vi "Dynamic call-Functional Viewer Window.vi"(8 "error in (no error)":errorcluster, 11 "Experiment data folder path":path) -> ()   [LabVIEW 2017]
uses:
  Globals/gl_Funct imaging UI.vi
panel:
  out "path":path
  # "Calls the \"Functional Viewer\" window dynamically."
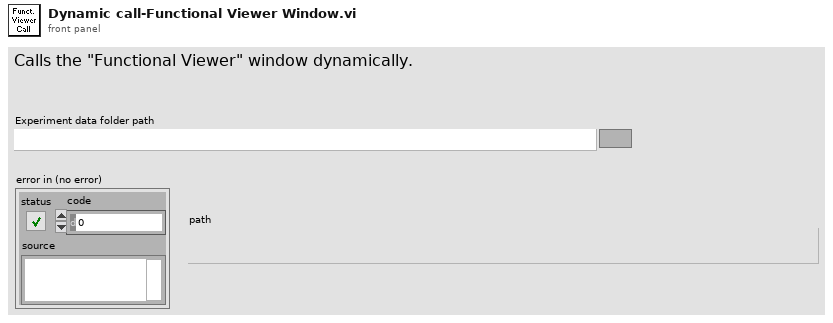
[diagram p1: front panel]
types:
  T1 = enum16{"Register", "Load dataset in funct viewer", "Re-process data"}
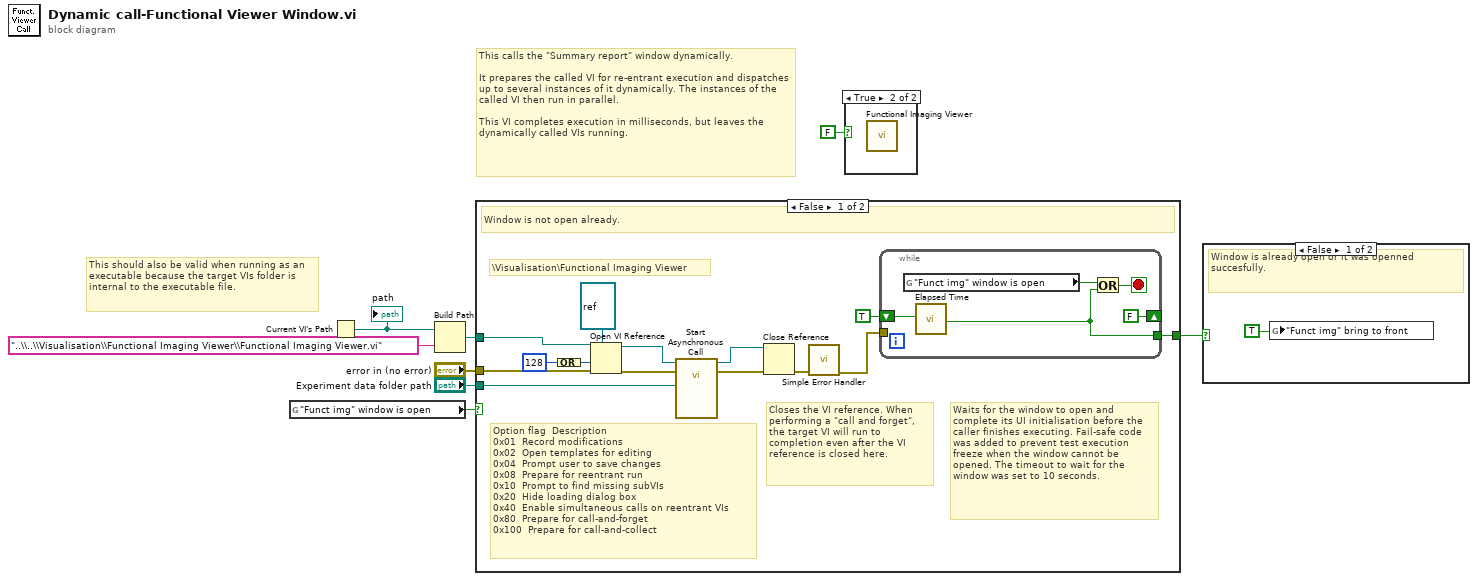
[diagram p0: block diagram]
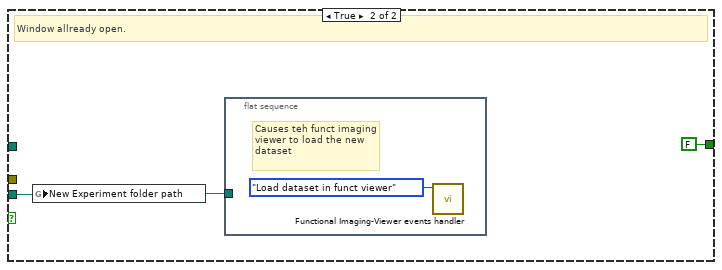
[diagram p4: hidden frame]
diagram:
  # "This should also be valid when running as an executable because the target VIs folder is internal to the executable file."
  # "This calls the \"Summary report\" window dynamically.\n\nIt prepares the called VI for re-entrant execution and dispatches up to several instances of it dynamically. The instances of the called VI then run in parallel.\n\nThis VI completes execution in milliseconds, but leaves the dynamically called VIs running."
  n1 = global read "gl_Funct imaging UI.vi" "\"Funct img\" window is open"() -> (w8:bool)
  n2 = Current VI's Path() -> (path=w4:path)
  "path" <- w4
  n3 = Build Path(base path=w4, name or relative path="..\\..\\Visualisation\\Functional Imaging Viewer\\Functional Imaging Viewer.vi") -> (appended path=w3:path)
  n4 = case shown="False" w8 {
    tunnel: "Experiment data folder path" -> [w12 w28]
    tunnel: "error in (no error)" -> [w11 _]
    tunnel: w3 -> [w10 _]
    tunnel: [w9 FALSE ("Time has Elapsed")] -> w1
    frame False {
      # "\\Visualisation\\Functional Imaging Viewer"
      # "Waits for the window to open and complete its UI initialisation before the caller finishes executing. Fail-safe code was added to prevent test execution freeze when the window cannot be opened. The timeout to wait for the window was set to 10 seconds."
      # "Option flag \tDescription\n0x01 \tRecord modifications\n0x02 \tOpen templates for editing\n0x04 \tPrompt user to save changes\n0x08 \tPrepare for reentrant run\n0x10 \tPrompt to find missing subVIs\n0x20 \tHide loading dialog box\n0x40 \tEnable simultaneous calls on reentrant VIs\n0x80 \tPrepare for call-and-forget\n0x100 \tPrepare for call-and-collect"
      # "Closes the VI reference. When performing a \"call and forget\", the target VI will run to completion even after the VI reference is closed here."
      # "Window is not open already."
      n5 = Compound Arithmetic op=OR(128) -> (w16:i32)
      n6 = Open VI Reference(type specifier VI Refnum (for type only)=refnum<vi> refnum, vi path=w10, options=w16, error in (no error)=w11) -> (vi reference=w15:refnum<vi>, error out=w14:errorcluster)  [unwired: 2 in]
      n7 = call-by-ref "Start Asynchronous Call"(reference=w15, error in=w14, "Experiment data folder path"=w12) -> (reference out=w21:refnum<vi>, error out=w20:errorcluster)  [unwired: 11 in]
      n8 = Close Reference(reference=w21, error in (no error)=w20) -> (error out=w22:errorcluster)
      n9 = call <vilib>:"Simple Error Handler.vi"("error in (no error)"=w22) -> ("error out"=w18:errorcluster)  [unwired: 4 in, 4 out]
      n10 = while {
        shift-right: [FALSE ("Reset")] -> _
        shift-left: TRUE ("Reset") -> [w26]
        tunnel: w18 -> [_]
        tunnel: [w23] -> w9
        stop <- w27 stop-if-true
        n11 = global read "gl_Funct imaging UI.vi" "\"Funct img\" window is open"() -> (w24:bool)
        n12 = call "Elapsed Time"("Reset"=w26) -> ("Time has Elapsed"=w23:bool)  [unwired: 11 in, 7 out]
        n13 = Or(x=w24, y=w23) -> (x .or. y?=w27:bool)
      }
    }
    frame True {
      # "Window allready open."
      n14 = global write "gl_Funct imaging UI.vi" "New Experiment folder path"(w28) -> ()
      n15 = flat-sequence {
        tunnel: w28 -> [_]
        frame #0 {
          # "Causes teh funct imaging viewer to load the new dataset"
          n16 = call "Functional Imaging-Viewer events handler.vi"("Event Function"=T1."Load dataset in funct viewer") -> ()  [unwired: 9 in, 2 out]
        }
      }
    }
  }
  n17 = case shown="True" FALSE {
    frame False {
    }
    frame True {
      n18 = call "Functional Imaging Viewer.vi"() -> ()  [unwired: 12 in]
    }
  }
  n19 = case shown="False" w1 {
    frame False {
      # "Window is already open or it was openned succesfully."
      n20 = global write "gl_Funct imaging UI.vi" "\"Funct img\" bring to front"(TRUE ("\"Values Check\" report window is open")) -> ()
    }
    frame True {
      # "Functional imaging viewer window failed to open"
    }
  }
